vi "U32 array to Base64.vi"(11 "Array":u32[](array[numeric])) -> (3 "Base64 sring out":string)   [LabVIEW 2020, in "wamplv.lvlib" / "Utils.lvclass"]
uses:
  Utils.lvclass
  Utils.lvclass/Utils.ctl
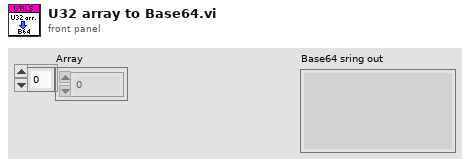
[diagram p1: front panel]
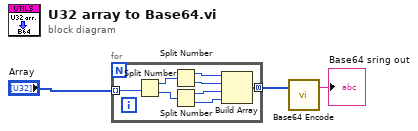
[diagram p0: block diagram]
diagram:
  n1 = for {
    tunnel: "Array" -> [w11] mode=indexing
    tunnel: [w4] -> w3 mode=concatenating
    n2 = Split Number(x=w11) -> (hi(x)=w10:u16, lo(x)=w9:u16)
    n3 = Split Number(x=w10) -> (hi(x)=w8:u8, lo(x)=w7:u8)
    n4 = Split Number(x=w9) -> (hi(x)=w6:u8, lo(x)=w5:u8)
    n5 = Build Array(w8, w7, w6, w5) -> (w4:u8[])
  }
  n6 = call "Base64 Encode.vi"("Bytes"=w3) -> ("Base64 sring out"=→"Base64 sring out":string)  [unwired: 2 in]
